vi "EnFlo_Tun_Heater_Control.vi"(1 "Ch Names":string[](array[string]), 2 "Values":dbl[](array[numeric]) format="%.2f") -> ()   [LabVIEW 2011]
uses:
  ADAM Client/Sub VIs/ADAM Controls/Search_mode.ctl
  ADAM_Global.vi
  <vilib>/Analysis/NI_AALPro.lvlib
  <vilib>/Analysis/NI_AALBase.lvlib
panel:
  in  "Total History":i32=80
  out "Proportional Term":dbl format="%#.1f"
  out "Control Sum":dbl format="%#.1f"
  out "Differential Term":dbl format="%#.1f"
  in  "Derivative History":i32=25
  out "Integral Term":dbl format="%#.1f"
  in  "Kp":dbl=2.0 format="%.2f"
  in  "Kd":dbl=10.0 format="%.2f"
  in  "Ki":dbl=0.05 format="%.2f"
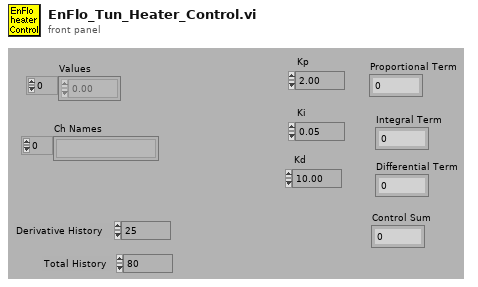
[diagram p1: front panel]
types:
  T1 = enum16{"On", "Off", "Always On", "Always Off", "Delete"}
  T2 = typedef "Search_mode.ctl" = enum16{"Between times", "All Times"}
  T3 = cluster{"Centre Times":dbl[], "Output array":dbl[]}
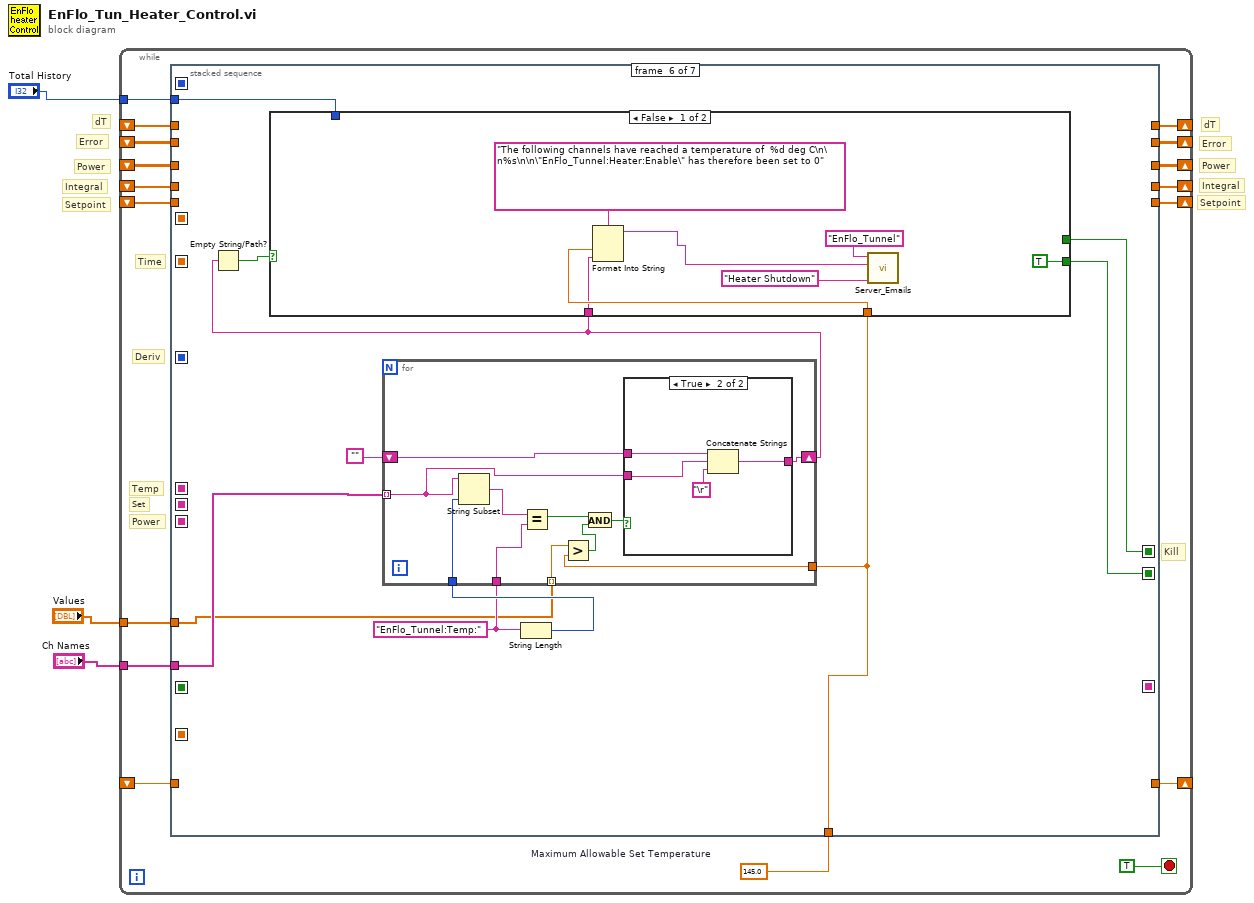
[diagram p0: block diagram]
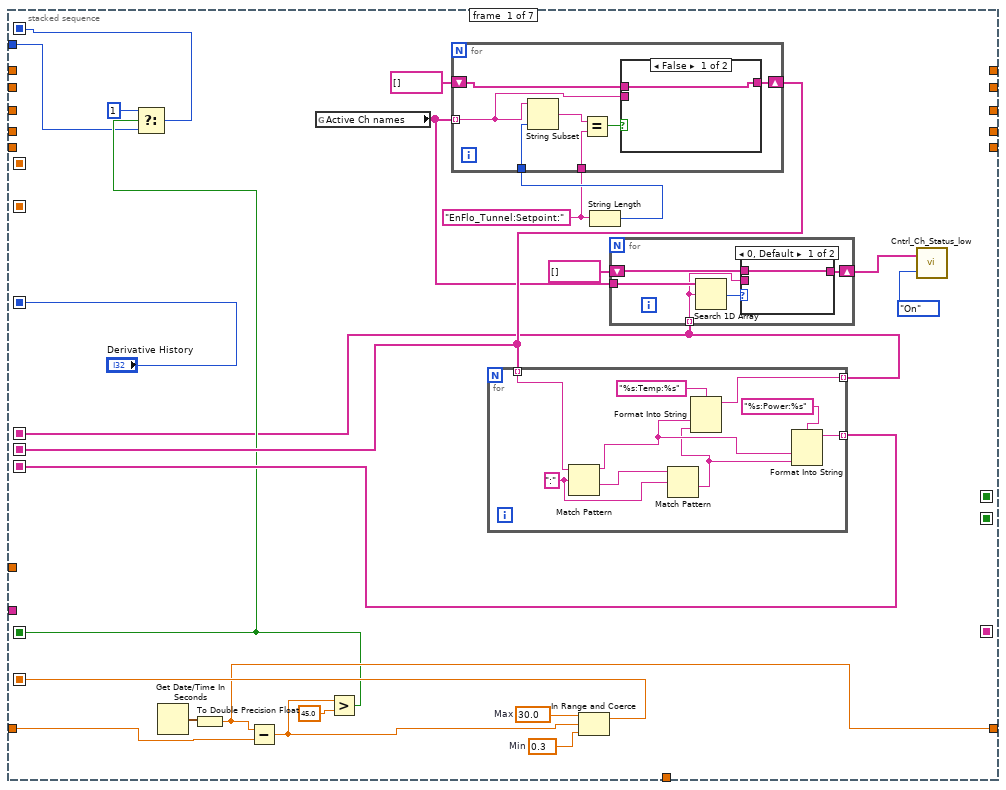
[diagram p2: hidden frame]
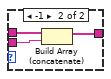
[diagram p3: hidden frame]
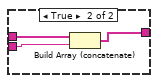
[diagram p4: hidden frame]
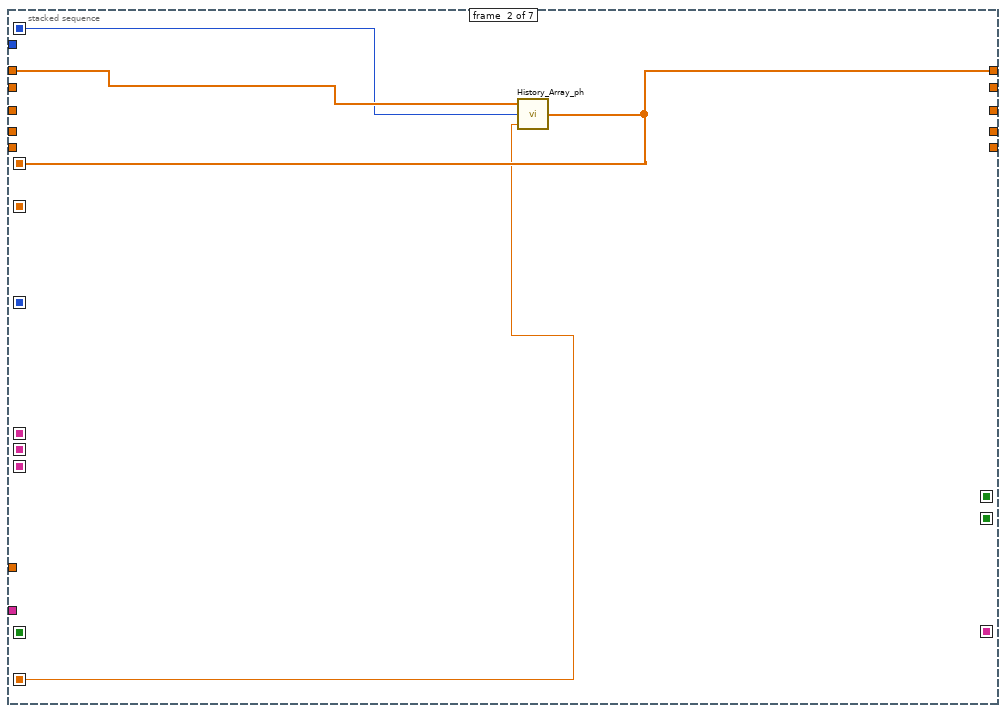
[diagram p5: hidden frame]
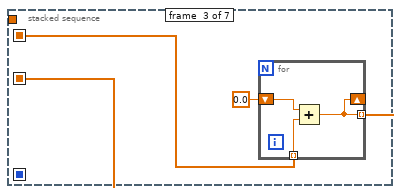
[diagram p6: hidden frame]
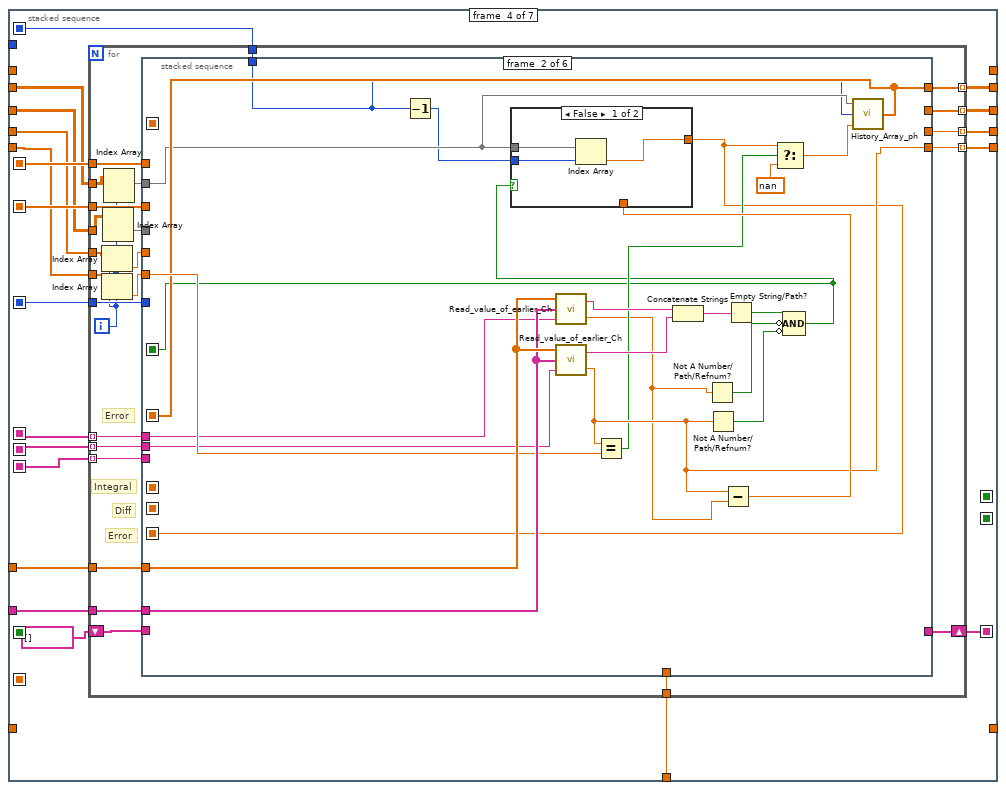
[diagram p7: hidden frame]
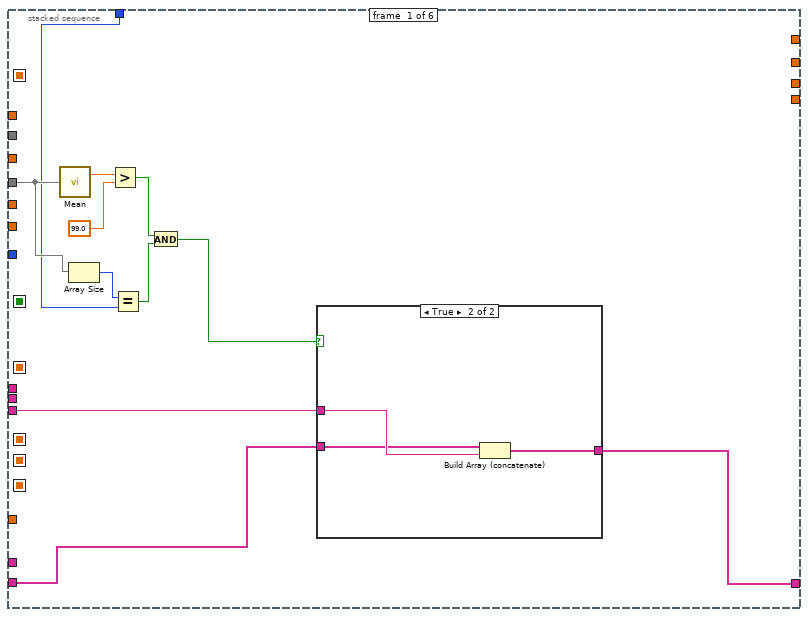
[diagram p8: hidden frame]
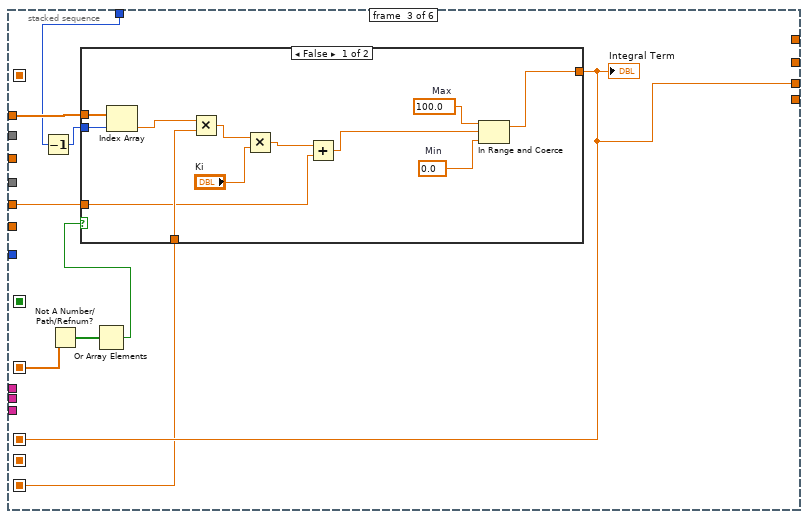
[diagram p11: hidden frame]
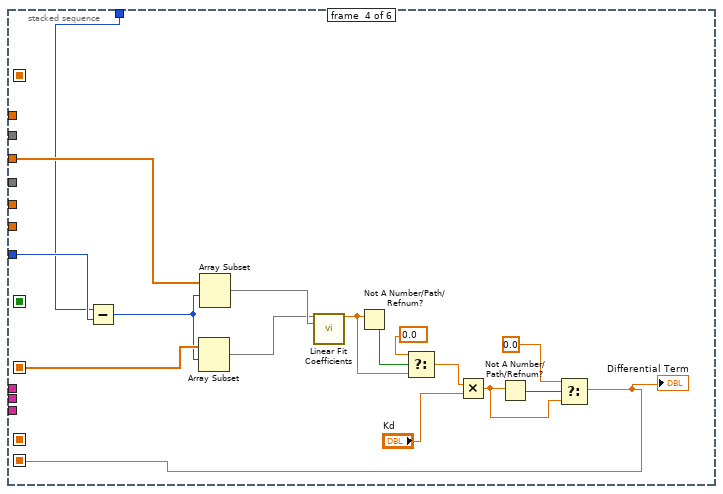
[diagram p13: hidden frame]
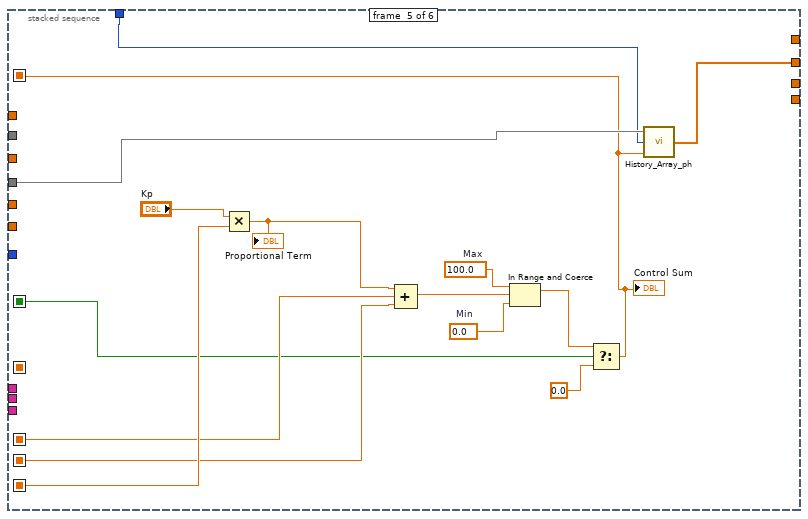
[diagram p14: hidden frame]
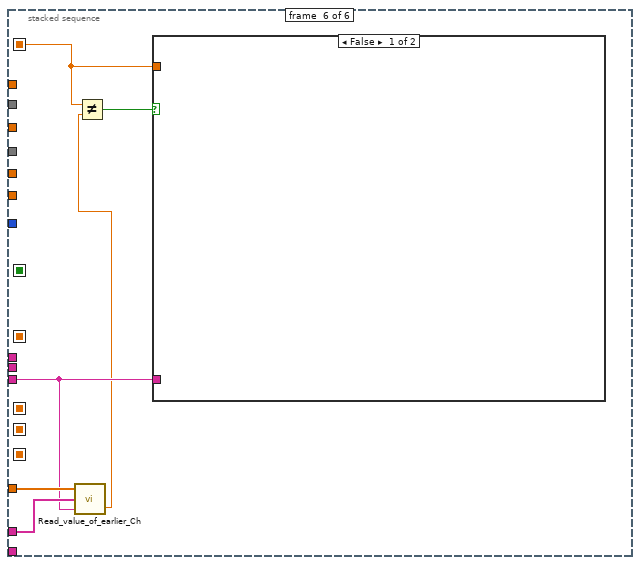
[diagram p15: hidden frame]
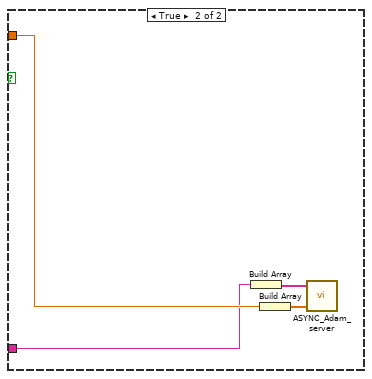
[diagram p16: hidden frame]
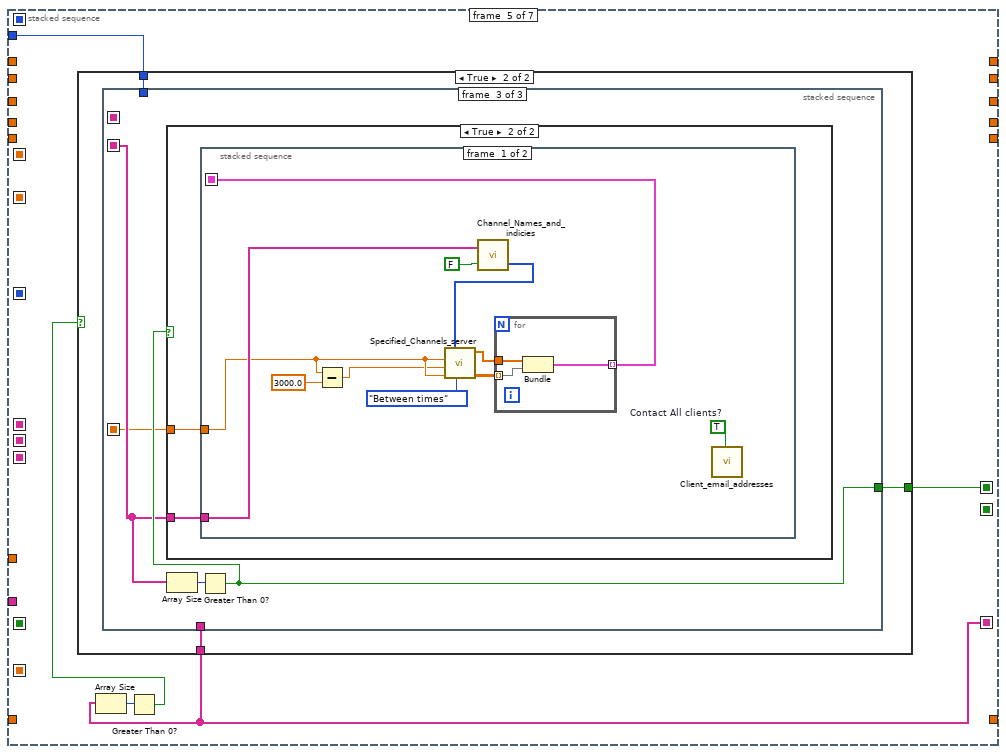
[diagram p17: hidden frame]
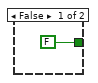
[diagram p18: hidden frame]
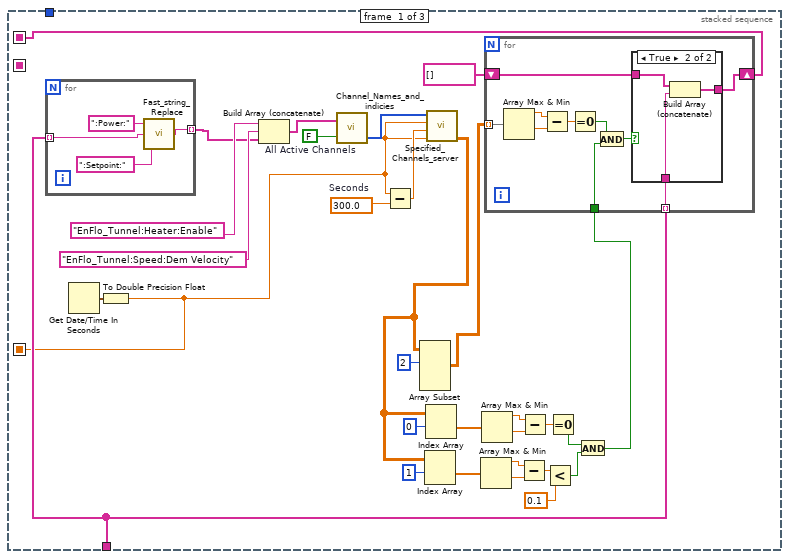
[diagram p19: hidden frame]
diagram:
  # "Setpoint"
  # "Integral"
  # "Power"
  # "Error"
  # "dT"
  # "Setpoint"
  # "Power"
  # "Integral"
  # "Error"
  # "dT"
  n1 = while {
    shift-right: [w18] -> _
    shift-left: _ -> [w19]
    shift-right: [w14] -> _
    shift-left: _ -> [w17]
    shift-right: [w16] -> _
    shift-left: _ -> [w15]
    shift-right: [w12] -> _
    shift-left: _ -> [w13]
    shift-right: [w10] -> _
    shift-left: _ -> [w11]
    shift-right: [w8] -> _
    shift-left: _ -> [w9]
    tunnel: "Total History" -> [w7]
    tunnel: "Ch Names" -> [w5]
    tunnel: "Values" -> [w4]
    stop <- TRUE stop-if-true
    w6 = 145.0  # Maximum Allowable Set Temperature
    # "Kill"
    # "Power"
    # "Set"
    # "Temp"
    # "Deriv"
    # "Time"
    n2 = stacked-sequence {
      seq-local: [_ w76 _ _ _ _ _] -> [_ _ w78 w101 _ _ _]
      seq-local: [_ _ w77 _ _ _ _] -> [_ _ _ w100 _ _ _]
      seq-local: ["Derivative History" _ _ _ _ _ _] -> [_ _ _ w96 _ _ _]
      seq-local: [w25 _ _ _ _ _ _] -> [_ _ _ w95 _ _ _]
      seq-local: [w40 _ _ _ _ _ _] -> [_ _ _ w94 _ _ _]
      seq-local: [w39 _ _ _ _ _ _] -> [_ _ _ w93 _ _ _]
      seq-local: [_ _ _ w90 _ _ _] -> [_ _ _ _ w235 _ _]
      seq-local: [_ _ _ _ w233 _ _] -> [_ _ _ _ _ w351 _]
      seq-local: [_ _ _ _ _ w352 _] -> [_ _ _ _ _ _ w378]
      seq-local: [w33 _ _ _ _ _ _] -> [_ w74 _ _ _ _ _]
      seq-local: [w29 _ _ _ _ _ _] -> [_ _ _ _ _ _ _]
      seq-local: [w27 _ _ _ _ _ _] -> [_ w73 _ w83 _ _ _]
      tunnel: w19 -> [_ w75 _ _ _ _ _]
      tunnel: [_ w76 _ _ _ _ _] -> w18
      tunnel: w17 -> [_ _ _ w87 _ _ _]
      tunnel: [w30 _ _ _ _ _ _] -> w16
      tunnel: w15 -> [w34 _ _ _ _ _ _]
      tunnel: [_ _ _ w102 _ _ _] -> w14
      tunnel: w13 -> [_ _ _ w86 _ _ _]
      tunnel: [_ _ _ w99 _ _ _] -> w12
      tunnel: w11 -> [_ _ _ w85 _ _ _]
      tunnel: [_ _ _ w98 _ _ _] -> w10
      tunnel: w9 -> [_ _ _ w84 _ _ _]
      tunnel: [_ _ _ w97 _ _ _] -> w8
      tunnel: w7 -> [w28 _ _ _ w236 w353 _]
      tunnel: w6 -> [_ _ _ w91 _ w345 _]
      tunnel: w5 -> [_ _ _ w89 _ w348 _]
      tunnel: w4 -> [_ _ _ w88 _ w347 _]
      frame #0 {
        w36 = 0.3  # Min
        w35 = 30.0  # Max
        w42 = "EnFlo_Tunnel:Setpoint:"
        n3 = Get Date/Time In Seconds() -> (seconds since 1Jan1904=w37:timestamp)
        n4 = To Double Precision Float(number=w37) -> (double precision float=w30:dbl)
        n5 = Subtract(x=w30, y=w34) -> (x-y=w32:dbl)
        n6 = global read "ADAM_Global.vi" "Active Ch names"() -> (w24:string[])
        n7 = Greater?(x=w32, y=45.0) -> (0:w29:bool)
        n8 = Select(t=1, s=w29, f=w28) -> (s? t:f=w27:i32)
        n9 = In Range and Coerce(upper limit=w35, x=w32, lower limit=w36) -> (coerced(x)=w33:dbl)  [unwired: 1 out]
        n10 = String Length(string=w42) -> (length=w43:i32)
        n11 = for {
          shift-right: [w53] -> w40
          shift-left: string[] [] -> [w55]
          tunnel: w24 -> [w54] mode=indexing
          tunnel: w43 -> [w59]
          tunnel: w42 -> [w58]
          n12 = String Subset(string=w54, length (rest)=w59) -> (substring=w57:string)  [unwired: 1 out]
          n13 = Equal?(x=w57, y=w58) -> (x = y?=w56:bool)
          n14 = case shown="False" w56 {
            tunnel: w55 -> [w60 w63]
            tunnel: w54 -> [_ w62]
            tunnel: [w60 w61] -> w53
            frame False {
            }
            frame True {
              n15 = Build Array (concatenate)(w63, w62) -> (w61:string[])
            }
          }
        }
        n16 = for {
          tunnel: w40 -> [w64] mode=indexing
          tunnel: [w65] -> w39 mode=indexing
          tunnel: [w66] -> w25 mode=indexing
          w71 = ":" ("regular expression")
          n17 = Match Pattern(string=w64, regular expression=w71) -> (before substring=w68:string, after substring=w72:string)  [unwired: 3 out]
          n18 = Match Pattern(string=w72, regular expression=w71) -> (after substring=w67:string)  [unwired: 4 out]
          n19 = Format Into String(format string="%s:Temp:%s", w68, w67) -> (resulting string=w66:string)  [unwired: 2 in, 1 out]
          n20 = Format Into String(format string="%s:Power:%s", w68, w67) -> (resulting string=w65:string)  [unwired: 2 in, 1 out]
        }
        n21 = for {
          shift-right: [w44] -> w21
          shift-left: string[] [] -> [w46]
          tunnel: w25 -> [w45] mode=indexing
          tunnel: w24 -> [w48]
          n22 = Search 1D Array(1D array=w48, element=w45) -> (index of element=w47:i32)  [unwired: 1 in]
          n23 = case shown="0, Default" w47 {
            tunnel: w46 -> [w49 w52]
            tunnel: w45 -> [_ w51]
            tunnel: [w49 w50] -> w44
            frame 0, Default {
            }
            frame -1 {
              n24 = Build Array (concatenate)(w52, w51) -> (w50:string[])
            }
          }
        }
        n25 = call "Cntrl_Ch_Status_low.vi"("Mode"=T1."On", "Channel names"=w21) -> ()  [unwired: 1 out]
      }
      frame #1 {
        n26 = call "History_Array_ph.vi"("Current Value"=w74, "Desired Length"=w73, "History In"=w75) -> ("History Out"=w76:dbl[])
      }
      frame #2 {
        n27 = for {
          shift-right: [w80] -> _
          shift-left: 0.0 ("element") -> [w82]
          tunnel: w78 -> [w81] mode=indexing
          tunnel: [w80] -> w77 mode=indexing
          n28 = Add(x=w82, y=w81) -> (x+y=w80:dbl)
        }
      }
      frame #3 {
        n29 = for {
          tunnel: w88 -> [w127]
          tunnel: w89 -> [w126]
          tunnel: [w125] -> w102 mode=indexing
          tunnel: w87 -> [w109]
          tunnel: w101 -> [w124]
          tunnel: w100 -> [w111]
          tunnel: [w123] -> w99 mode=indexing
          tunnel: w86 -> [w110]
          tunnel: [w122] -> w98 mode=indexing
          tunnel: w85 -> [w112]
          tunnel: [w121] -> w97 mode=indexing
          tunnel: w84 -> [w106]
          tunnel: w96 -> [w120]
          tunnel: w95 -> [w119] mode=indexing
          tunnel: w94 -> [w118] mode=indexing
          tunnel: w93 -> [w117] mode=indexing
          shift-right: [w115] -> w90
          shift-left: string[] [] -> [w116]
          tunnel: w91 -> [w114]
          tunnel: w83 -> [w103]
          i -> [w104]
          # "Integral"
          # "Error"
          # "Error"
          # "Diff"
          n30 = Index Array(array=w112, index=w104) -> (element=w113:dbl)
          n31 = Index Array(array=w106, index=w104) -> (element=w105:dbl)
          n32 = Index Array(array=w110, index (row)=w104) -> (element=w107:dbl[])  [unwired: 1 in]
          n33 = Index Array(array=w109, index (row)=w104) -> (element=w108:dbl[])  [unwired: 1 in]
          n34 = stacked-sequence {
            seq-local: [_ _ _ w201 _ _] -> [_ _ _ _ w218 _]
            seq-local: [_ w153 _ _ _ _] -> [_ _ w176 _ w222 _]
            seq-local: [_ w148 _ _ _ _] -> [_ _ w174 w196 _ _]
            seq-local: [_ _ w178 _ _ _] -> [_ _ _ _ w219 _]
            seq-local: [_ _ _ _ w209 _] -> [_ _ _ _ _ w227]
            seq-local: [_ w143 _ _ _ _] -> [_ _ _ _ w211 _]
            tunnel: w127 -> [_ w165 _ _ _ w226]
            tunnel: w126 -> [_ w164 _ _ _ w225]
            tunnel: [_ w148 _ _ _ _] -> w125
            tunnel: w108 -> [_ w147 _ _ _ _]
            tunnel: w124 -> [_ _ w177 _ _ _]
            tunnel: w111 -> [_ _ _ w198 _ _]
            tunnel: [_ _ _ _ w214 _] -> w123
            tunnel: w107 -> [w136 _ _ _ w213 _]
            tunnel: [_ _ w178 _ _ _] -> w122
            tunnel: w113 -> [_ _ w175 _ _ _]
            tunnel: [_ w156 _ _ _ _] -> w121
            tunnel: w105 -> [_ w155 _ _ _ _]
            tunnel: w120 -> [_ _ _ w193 _ _]
            tunnel: w119 -> [_ w149 _ _ _ _]
            tunnel: w118 -> [_ w151 _ _ _ _]
            tunnel: w117 -> [w131 _ _ _ _ w224]
            tunnel: w116 -> [w130 _ _ _ _ _]
            tunnel: [w129 _ _ _ _ _] -> w115
            tunnel: w114 -> [_ _ _ _ _ _]
            tunnel: w103 -> [w128 w145 w171 w192 w212 _]
            frame #0 {
              n35 = call <vilib>:"Mean.vi"("X"=w136) -> ("mean"=w138:dbl)  [unwired: 1 out]
              n36 = Array Size(array=w136) -> (size(s)=w135:i32)
              n37 = Greater?(x=w138, y=99.0) -> (0:w133:bool)
              n38 = Equal?(x=w135, y=w128) -> (x = y?=w134:bool)
              n39 = And(x=w133, y=w134) -> (x .and. y?=w132:bool)
              n40 = case shown="True" w132 {
                tunnel: w131 -> [_ w142]
                tunnel: w130 -> [w139 w141]
                tunnel: [w139 w140] -> w129
                frame False {
                }
                frame True {
                  n41 = Build Array (concatenate)(w141, w142) -> (w140:string[])
                }
              }
            }
            frame #1 {
              n42 = Decrement(x=w145) -> (x-1=w144:i32)
              n43 = call "Read_value_of_earlier_Ch.vi"("Desired Ch to Read"=w149, "Ch names"=w164, "Present scan array"=w165) -> ("Value"=w150:dbl, "Scan comment"=w163:string)  [unwired: 1 in]
              n44 = call "Read_value_of_earlier_Ch.vi"("Desired Ch to Read"=w151, "Ch names"=w164, "Present scan array"=w165) -> ("Value"=w156:dbl, "Scan comment"=w162:string)  [unwired: 1 in]
              n45 = Equal?(x=w156, y=w155) -> (x = y?=w154:bool)
              n46 = Concatenate Strings(w163, w162) -> (w161:string)
              n47 = Not A Number/Path/Refnum?(number/path/refnum=w150) -> (NaN/Path/Refnum?=w159:bool)
              n48 = Not A Number/Path/Refnum?(number/path/refnum=w156) -> (NaN/Path/Refnum?=w158:bool)
              n49 = Subtract(x=w156, y=w150) -> (x-y=w157:dbl)
              n50 = Empty String/Path?(string/path=w161) -> (empty?=w160:bool)
              n51 = Compound Arithmetic op=AND(w160, invert w159, invert w158) -> (w143:bool)
              n52 = case shown="False" w143 {
                tunnel: w144 -> [w168 _]
                tunnel: w147 -> [w167 _]
                tunnel: [w166 w169] -> w153
                tunnel: w157 -> [_ w169]
                frame False {
                  n53 = Index Array(array=w167, index=w168) -> (element=w166:dbl)
                }
                frame True {
                }
              }
              n54 = Select(t=w153, s=w154, f=nan) -> (s? t:f=w146:dbl)
              n55 = call "History_Array_ph.vi"("Current Value"=w146, "Desired Length"=w145, "History In"=w147) -> ("History Out"=w148:dbl[])
            }
            frame #2 {
              n56 = Decrement(x=w171) -> (x-1=w170:i32)
              n57 = Not A Number/Path/Refnum?(number/path/refnum=w174) -> (NaN/Path/Refnum?=w173:bool[])
              n58 = Or Array Elements(Boolean array=w173) -> (logical OR=w172:bool)
              n59 = case shown="False" w172 {
                tunnel: [w187 w191] -> w178
                tunnel: w170 -> [w186 _]
                tunnel: w177 -> [w185 _]
                tunnel: w176 -> [w183 _]
                tunnel: w175 -> [w181 w191]
                frame False {
                  w190 = 0.0  # Min
                  w188 = 100.0  # Max
                  n60 = Index Array(array=w185, index=w186) -> (element=w184:dbl)
                  n61 = Multiply(x=w184, y=w183) -> (x*y=w182:dbl)
                  n62 = Multiply(x=w182, y="Ki") -> (x*y=w180:dbl)
                  n63 = Add(x=w180, y=w181) -> (x+y=w179:dbl)
                  n64 = In Range and Coerce(upper limit=w188, x=w179, lower limit=w190) -> (coerced(x)=w187:dbl)  [unwired: 1 out]
                }
                frame True {
                }
              }
              "Integral Term" <- w178
            }
            frame #3 {
              n65 = Subtract(x=w192, y=w193) -> (x-y=w194:i32)
              n66 = Array Subset(array=w196, index=w194) -> (w195:dbl[])  [unwired: 1 in]
              n67 = Array Subset(array=w198, index=w194) -> (w197:dbl[])  [unwired: 1 in]
              n68 = call <vilib>:"Linear Fit Coefficients.vi"("Y"=w195, "X"=w197) -> ("slope"=w207:dbl)  [unwired: 3 in, 10 out]
              n69 = Not A Number/Path/Refnum?(number/path/refnum=w207) -> (NaN/Path/Refnum?=w205:bool)
              n70 = Select(t=0.0 ("f"), s=w205, f=w207) -> (s? t:f=w204:dbl)
              n71 = Multiply(x=w204, y="Kd") -> (x*y=w200:dbl)
              n72 = Not A Number/Path/Refnum?(number/path/refnum=w200) -> (NaN/Path/Refnum?=w202:bool)
              n73 = Select(t=0.0, s=w202, f=w200) -> (s? t:f=w201:dbl)
              "Differential Term" <- w201
            }
            frame #4 {
              w217 = 0.0  # Min
              w216 = 100.0  # Max
              n74 = Multiply(x="Kp", y=w222) -> (x*y=w220:dbl)
              "Proportional Term" <- w220
              n75 = Compound Arithmetic op=ADD(w220, w219, w218) -> (w215:dbl)
              n76 = In Range and Coerce(upper limit=w216, x=w215, lower limit=w217) -> (coerced(x)=w210:dbl)  [unwired: 1 out]
              n77 = Select(t=w210, s=w211, f=0.0) -> (s? t:f=w209:dbl)
              "Control Sum" <- w209
              n78 = call "History_Array_ph.vi"("Current Value"=w209, "Desired Length"=w212, "History In"=w213) -> ("History Out"=w214:dbl[])
            }
            frame #5 {
              n79 = call "Read_value_of_earlier_Ch.vi"("Desired Ch to Read"=w224, "Ch names"=w225, "Present scan array"=w226) -> ("Value"=w223:dbl)  [unwired: 1 in, 1 out]
              n80 = Not Equal?(x=w227, y=w223) -> (x != y?=w228:bool)
              n81 = case shown="False" w228 {
                tunnel: w227 -> [_ w230]
                tunnel: w224 -> [_ w229]
                frame False {
                }
                frame True {
                  n82 = Build Array(w229) -> (w231:string[])
                  n83 = Build Array(w230) -> (w232:dbl[])
                  n84 = call "ASYNC_Adam_server.vi"("Values"=w232, "Channel Names"=w231) -> ()  [unwired: 1 in, 3 out]
                }
              }
            }
          }
        }
      }
      frame #4 {
        n85 = Array Size(array=w235) -> (size(s)=w237:i32)
        n86 = Greater Than 0?(x=w237) -> (x > 0?=w234:bool)
        n87 = case shown="True" w234 {
          tunnel: w236 -> [_ w240]
          tunnel: w235 -> [_ w241]
          tunnel: [FALSE w239] -> w233
          frame False {
          }
          frame True {
            n88 = stacked-sequence {
              seq-local: [w266 _ _] -> [_ w291 _]
              seq-local: [w242 _ _] -> [_ w297 w310]
              seq-local: [_ w292 _] -> [_ _ w311]
              tunnel: w241 -> [w265 _ _]
              tunnel: w240 -> [_ _ _]
              tunnel: [_ _ w312] -> w239
              frame #0 {
                w269 = 300.0  # Seconds
                w271 = FALSE  # All Active Channels
                n89 = for {
                  tunnel: w265 -> [w287] mode=indexing
                  tunnel: [w286] -> w243 mode=indexing
                  n90 = call "Fast_string_Replace.vi"("Replace match with:"=":Setpoint:" ("regular expression"), "Input String"=w287, "regular expression"=":Power:") -> ("Output String"=w286:string)  [unwired: 2 out]
                }
                n91 = Get Date/Time In Seconds() -> (seconds since 1Jan1904=w268:timestamp)
                n92 = To Double Precision Float(number=w268) -> (double precision float=w242:dbl)
                n93 = Build Array (concatenate)("EnFlo_Tunnel:Heater:Enable", "EnFlo_Tunnel:Speed:Dem Velocity", w243) -> (w262:string[])
                n94 = call "Channel_Names_and_indicies.vi"("All Active Channels"=w271, "Desired Ch Names"=w262) -> ("Indicies"=w270:i32[])  [unwired: 1 out]
                n95 = Subtract(x=w242, y=w269) -> (x-y=w264:dbl)
                n96 = call "Specified_Channels_server.vi"("End time"=w242, "Start time"=w264, "Clients time"=w242, "Requested channels"=w270) -> ("Output array"=w249:dbl[][])  [unwired: 1 in, 4 out]
                n97 = Array Subset(array=w249, index (row)=2 ("index")) -> (w260:dbl[][])  [unwired: 3 in]
                n98 = Index Array(array=w249, index (row)=1) -> (element=w254:dbl[])  [unwired: 1 in]
                n99 = Index Array(array=w249, index (row)=0) -> (element=w256:dbl[])  [unwired: 1 in]
                n100 = Array Max & Min(array=w254) -> (max value=w252:dbl, min value=w253:dbl)  [unwired: 2 out]
                n101 = Array Max & Min(array=w256) -> (max value=w258:dbl, min value=w257:dbl)  [unwired: 2 out]
                n102 = Subtract(x=w252, y=w253) -> (x-y=w246:dbl)
                n103 = Subtract(x=w258, y=w257) -> (x-y=w259:dbl)
                n104 = Less?(x=w246, y=0.1) -> (x < y?=w244:bool)
                n105 = Equal To 0?(x=w259) -> (x = 0?=w248:bool)
                n106 = And(x=w248, y=w244) -> (x .and. y?=w247:bool)
                n107 = for {
                  tunnel: w260 -> [w281] mode=indexing
                  shift-right: [w275] -> w266
                  shift-left: string[] [] -> [w276]
                  tunnel: w265 -> [w277] mode=indexing
                  tunnel: w247 -> [w272]
                  n108 = Array Max & Min(array=w281) -> (max value=w279:dbl, min value=w280:dbl)  [unwired: 2 out]
                  n109 = Subtract(x=w279, y=w280) -> (x-y=w278:dbl)
                  n110 = Equal To 0?(x=w278) -> (x = 0?=w274:bool)
                  n111 = And(x=w274, y=w272) -> (x .and. y?=w273:bool)
                  n112 = case shown="True" w273 {
                    tunnel: w277 -> [_ w285]
                    tunnel: w276 -> [w282 w284]
                    tunnel: [w282 w283] -> w275
                    frame False {
                    }
                    frame True {
                      n113 = Build Array (concatenate)(w284, w285) -> (w283:string[])
                    }
                  }
                }
              }
              frame #1 {
                n114 = Subtract(x=w297, y=320.0) -> (x-y=w298:dbl)
                n115 = call "Get_ADAM_averages_server.vi"("No of averages"=1, "End time"=w297, "Start time"=w298, "Clients time"=w297, "ADAM Ch Names"=w291) -> ("DBL values"=w295:dbl[][])  [unwired: 1 in, 4 out]
                n116 = Index Array(array=w295, index (row)=0) -> (element=w293:dbl[])  [unwired: 1 in]
                n117 = for {
                  shift-right: [w304] -> w292
                  shift-left: string[] [] -> [w300]
                  tunnel: w291 -> [w305] mode=indexing
                  tunnel: w293 -> [w303] mode=indexing
                  n118 = Greater?(x=w303, y=99.0) -> (0:w301:bool)
                  n119 = case shown="True" w301 {
                    tunnel: w305 -> [_ w309]
                    tunnel: w300 -> [w306 w308]
                    tunnel: [w306 w307] -> w304
                    frame False {
                    }
                    frame True {
                      n120 = Build Array (concatenate)(w308, w309) -> (w307:string[])
                    }
                  }
                }
              }
              frame #2 {
                n121 = Array Size(array=w311) -> (size(s)=w313:i32)
                n122 = Greater Than 0?(x=w313) -> (x > 0?=w312:bool)
                n123 = case shown="True" w312 {
                  tunnel: w311 -> [_ w315]
                  tunnel: w310 -> [_ w314]
                  frame False {
                  }
                  frame True {
                    n124 = stacked-sequence {
                      seq-local: [w317 _] -> [_ w331]
                      tunnel: w315 -> [w322 w333]
                      tunnel: w314 -> [w321 _]
                      frame #0 {
                        w316 = TRUE  # Contact All clients?
                        n125 = Subtract(x=w321, y=3000.0) -> (x-y=w319:dbl)
                        n126 = call "Channel_Names_and_indicies.vi"("All Active Channels"=FALSE, "Desired Ch Names"=w322) -> ("Indicies"=w325:i32[])  [unwired: 1 out]
                        n127 = call "Specified_Channels_server.vi"("Mode"=Search_mode."Between times", "End time"=w321, "Start time"=w319, "Clients time"=w321, "Requested channels"=w325) -> ("Output array"=w318:dbl[][], "Centre Times"=w326:dbl[])  [unwired: 3 out]
                        n128 = for {
                          tunnel: w326 -> [w329]
                          tunnel: w318 -> [w328] mode=indexing
                          tunnel: [w327] -> w317 mode=indexing
                          n129 = Bundle("Centre Times"=w329, "Output array"=w328) -> (w327:T3)  [unwired: 1 out]
                        }
                        n130 = call "Client_email_addresses.vi"("Contact All clients?"=w316) -> ()  [unwired: 2 in]
                      }
                      frame #1 {
                        n131 = for {
                          shift-right: [w339] -> w337
                          shift-left: "" -> [w342]
                          tunnel: w333 -> [w340] mode=indexing
                          n132 = Concatenate Strings(w342, w340, "\r") -> (w339:string)
                        }
                        n133 = Format Into String(format string="The following channels have been at 100%% Power for 5 minutes\n\n%s\n\n\"EnFlo_Tunnel:Heater:Enable\" has therefore been set to 0", w337) -> (resulting string=w334:string)  [unwired: 2 in, 1 out]
                        n134 = call "Email_Attachment_Plot.vi"("X axis name"="Time", "Y axis name"="Power (%)", "XY Graph"=w331, "Series Names"=w333, "message"=w334, "subject ([No Subject])"="Heater Shutdown" ("t")) -> ()  [unwired: 1 out]
                      }
                    }
                  }
                }
              }
            }
          }
        }
      }
      frame #5 {
        w349 = "EnFlo_Tunnel:Temp:"
        n135 = String Length(string=w349) -> (length=w350:i32)
        n136 = for {
          shift-right: [w359] -> w343
          shift-left: "" -> [w360]
          tunnel: w348 -> [w363] mode=indexing
          tunnel: w350 -> [w364]
          tunnel: w349 -> [w361]
          tunnel: w347 -> [w358] mode=indexing
          tunnel: w345 -> [w357]
          n137 = String Subset(string=w363, length (rest)=w364) -> (substring=w362:string)  [unwired: 1 out]
          n138 = Equal?(x=w362, y=w361) -> (x = y?=w354:bool)
          n139 = Greater?(x=w358, y=w357) -> (0:w355:bool)
          n140 = And(x=w354, y=w355) -> (x .and. y?=w356:bool)
          n141 = case shown="True" w356 {
            tunnel: w363 -> [_ w366]
            tunnel: w360 -> [w365 w368]
            tunnel: [w365 w367] -> w359
            frame False {
            }
            frame True {
              n142 = Concatenate Strings(w368, w366, "\r") -> (w367:string)
            }
          }
        }
        n143 = Empty String/Path?(string/path=w343) -> (empty?=w344:bool)
        n144 = case shown="False" w344 {
          tunnel: w353 -> [_ _]
          tunnel: w345 -> [w371 _]
          tunnel: [TRUE w377] -> w352
          tunnel: w351 -> [_ w377]
          tunnel: w343 -> [w370 _]
          frame False {
            n145 = Format Into String(format string="The following channels have reached a temperature of  %d deg C\n\n%s\n\n\"EnFlo_Tunnel:Heater:Enable\" has therefore been set to 0", w371, w370) -> (resulting string=w373:string)  [unwired: 2 in, 1 out]
            n146 = call "Server_Emails.vi"("Client Name Contains"="EnFlo_Tunnel", "Message"=w373, "Subject"="Heater Shutdown" ("t")) -> ()  [unwired: 2 in, 3 out]
          }
          frame True {
          }
        }
      }
      frame #6 {
        n147 = case shown="True" w378 {
          frame False {
          }
          frame True {
            n148 = Build Array("EnFlo_Tunnel:Heater:Enable") -> (w381:string[])
            n149 = Build Array(0.0) -> (w379:dbl[])
            n150 = call "ASYNC_Adam_server.vi"("Values"=w379, "Channel Names"=w381) -> ()  [unwired: 1 in, 3 out]
          }
        }
      }
    }
  }
